vi "ActorLightRun.vi"(8 "ErrorIn":errorcluster, 11 "YActorIn":refnum<class "YActor.lvclass">) -> (0 "ErrorOut":errorcluster, 3 "YActorOut":refnum<class "YActor.lvclass">)   [LabVIEW 2021, in "YActor.lvclass"]
uses:
  YActor.lvclass
  <vilib>/Utility/miscctls.llb/LVPointTypeDef.ctl
  private/ActorPoolFunctions.ctl
  YActor.lvclass/YActor.ctl
  private/GetVIRef.vi
  private/BinaryTracer.vi
  Prefix error msg.vi
  Debug Messages.vi
  private/VIMethodTemplate.vi
  private/RawTrace.vi
panel:
  in  "GuiRef":refnum<vi>
  out "Top Level":string
  in  "LogHistory":u32=30
  out "CommandHistory":string[](array[string])
  in  "KeepOpen":bool
  out "Time Stamp":timestamp format="%<%x %.3X>T"
  in  "SingleStep":bool
  out "Data":string
  out "Command":string
  in  "Continue":bool
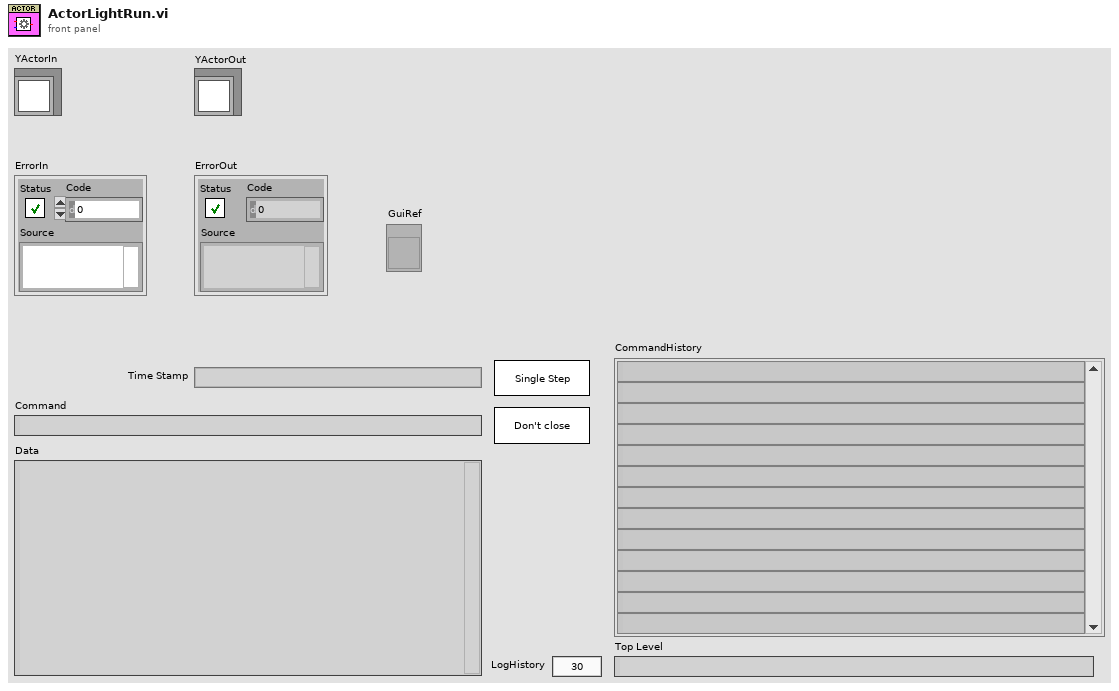
[diagram p1: front panel]
types:
  T1 = typedef "YActor.lvclass/ActorPoolFunctions.ctl" = enum16{"Add", "GetAll", "Delete"}
  T2 = typedef "LVPointTypeDef.ctl" = cluster{"Horizontal":i16, "Vertical":i16}
  T3 = typedef "YActor.lvclass/CmdCtrl.ctl" = cluster{"CmdData":variant, "CommandVI":string, "ReplyQ":i64, "Error":errorcluster, "Msg#":u32, "AsyncErrorHandling":T4, "CallMode":T5, "Source":string}
  T4 = typedef "YActor.lvclass/AsyncErrorHandling.ctl" = enum16{"Return after executing sync command", "Return before executing sync command", "Don't return error"}
  T5 = typedef "YActor.lvclass/CallMode.ctl" = enum16{"Standard", "Call&Collect"}
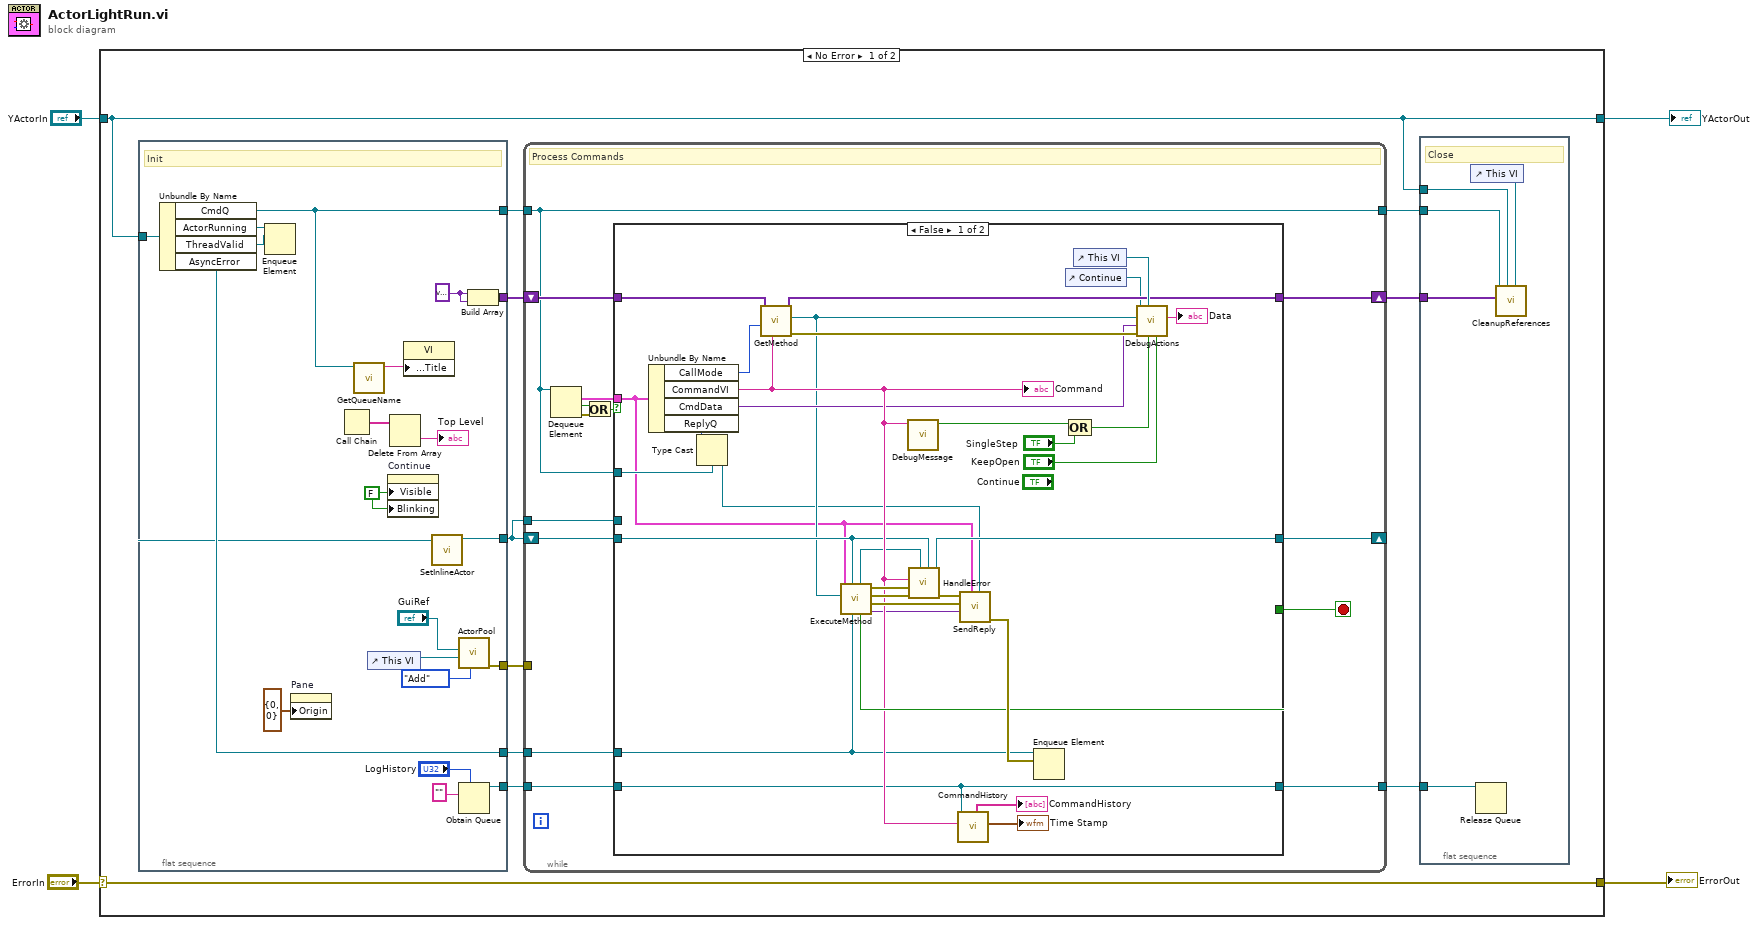
[diagram p0: block diagram]
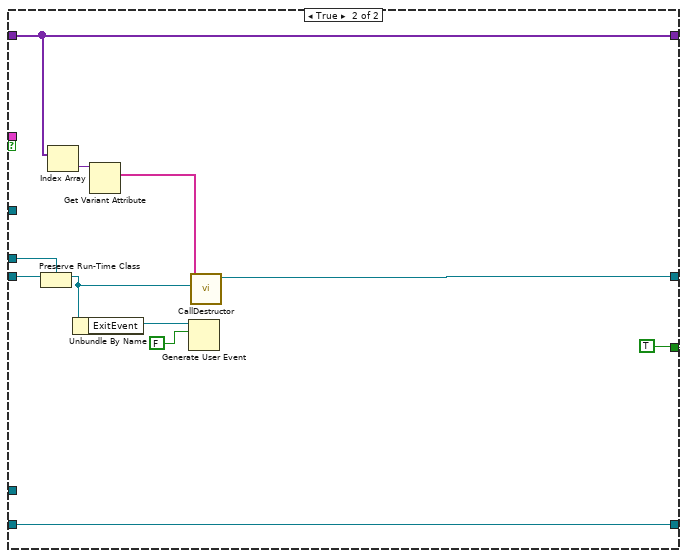
[diagram p2: hidden frame]
diagram:
  n1 = case shown="No Error" "ErrorIn" {
    selector: "ErrorIn" -> [w15 w99]
    tunnel: [w15 w99] -> w3
    tunnel: [w6 w98] -> w1
    tunnel: "YActorIn" -> [w6 w98]
    frame No Error {
      n2 = flat-sequence {
        tunnel: [w21] -> w13
        tunnel: [w37] -> w12
        tunnel: [w35] -> w11
        tunnel: [w29] -> w5
        tunnel: [w27] -> w10
        tunnel: [w40] -> w14
        tunnel: w6 -> [w22]
        frame #0 {
          w28 = variant
          w38 = FALSE ("Visible")
          # "Init"
          n3 = Unbundle By Name(w22) -> ("CmdQ"=w21:refnum<queue>, "ActorRunning"=w33:refnum<queue>, "ThreadValid"=w32:refnum<queue>, "AsyncError"=w27:refnum<queue>)
          n4 = Enqueue Element(queue=w33, element=w32) -> ()  [unwired: 2 in, 3 out]
          n5 = property on="Pane" class="Pane"("Origin"=T2 {"Horizontal"=0, "Vertical"=0}) -> ()  [unwired: 2 in, 2 out]
          n6 = Call Chain() -> (call chain=w31:string[])
          n7 = call "GetQueueName.vi"("QueueIn"=w21) -> ("String"=w26:string)  [unwired: 10 in]
          n8 = control-ref of="This VI"() -> (w24:refnum<vi>)
          n9 = property on="Continue" class="Bool"("Visible"=w38, "Blinking"=w38) -> ()  [unwired: 2 in, 2 out]
          n10 = Delete From Array(array=w31) -> (deleted portion=→"Top Level":string)  [unwired: 2 in, 1 out]
          n11 = property class="VI"("Front Panel.Title"=w26) -> ()  [unwired: 2 in, 2 out]
          n12 = call "SetInlineActor.vi"("YActorIn"=w22) -> ("YActorOut"=w29:refnum<class "YActor.lvclass">)  [unwired: 9 in, 1 out]
          n13 = call "ActorPool.vi"("Functions"=ActorPoolFunctions."Add", "ActorRef"=w24, "GuiRef"="GuiRef") -> ("ErrorOut"=w40:errorcluster)  [unwired: 6 in, 2 out]
          n14 = Obtain Queue(max queue size (-1, unlimited)="LogHistory", element data type="") -> (queue out=w35:refnum<queue>)  [unwired: 3 in, 2 out]
          n15 = Build Array(w28, w28) -> (w37:variant[])
        }
      }
      n16 = while {
        shift-right: [w51] -> w8
        shift-left: w12 -> [w52]
        shift-right: [w50] -> _
        shift-left: w5 -> [w49]
        tunnel: [w41] -> w9
        tunnel: w13 -> [w41]
        tunnel: w11 -> [w45]
        tunnel: w10 -> [w44]
        tunnel: w5 -> [w43]
        tunnel: [w42] -> w7
        tunnel: w14 -> [_]
        stop <- w46 stop-if-true
        # "Process Commands"
        n17 = Dequeue Element(queue=w41) -> (element=w53:T3, timed out?=w48:bool, error out=w54:errorcluster)  [unwired: 2 in, 1 out]
        n18 = Or(x=w48, y=w54) -> (x .or. y?=w47:bool)
        n19 = case shown="False" w47 {
          tunnel: w53 -> [w56 _]
          tunnel: w52 -> [w66 w96]
          tunnel: [w65 w96] -> w51
          tunnel: w41 -> [w80 _]
          tunnel: [w74 w94] -> w50
          tunnel: w49 -> [w61 w95]
          tunnel: [w75 TRUE] -> w46
          tunnel: w45 -> [w57 w87]
          tunnel: w44 -> [w58 _]
          tunnel: w43 -> [_ w93]
          tunnel: [w57 w87] -> w42
          frame False {
            n20 = Unbundle By Name(w56) -> ("CallMode"=w70:T5, "CommandVI"=w71:string, "CmdData"=w63:variant, "ReplyQ"=w79:i64)
            "Command" <- w71
            n21 = Type Cast(type=w80, x=w79) -> (*(type *) &x=w55:refnum<queue>)
            n22 = call "GetMethod.vi"("CommandVI"=w71, "CallMode"=w70, "ReferencesIn"=w66) -> ("ErrorOut"=w86:errorcluster, "VIOut"=w59:refnum<vi>, "ReferencesOut"=w65:variant[])  [unwired: 6 in]
            n23 = call "ExecuteMethod.vi"("AsyncError"=w58, "LabVIEWObjectIn"=w61, "VIIn"=w59, "QueueDataIn"=w56) -> ("ReplyData"=w60:variant, "AsyncErrorOut"=w81:errorcluster, "MethodErrorOut"=w83:errorcluster, "VICallErrorOut"=w84:errorcluster, "Exit"=w75:bool, "LabVIEWObjectOut"=w62:refnum<class>)  [unwired: 2 in]
            n24 = call "DebugMessage.vi"("CommandVI"=w71) -> ("StartDebug"=w76:bool)  [unwired: 10 in]
            n25 = call "HandleError.vi"("LabVIEWObjectIn"=w61, "MethodDataOutput"=w62, "ErrorIn"=w83, "VICallError"=w84, "CommandVI"=w71) -> ("ErrorOut"=w82:errorcluster, "MethodDataOutput"=w74:refnum<class>)  [unwired: 5 in]
            n26 = call "CommandHistory.vi"("CommandVI"=w71, "QueueIn"=w57) -> ("SecondsSince1Jan1904"=→"Time Stamp":timestamp, "HiStory"=→"CommandHistory":string[])  [unwired: 8 in]
            n27 = call "SendReply.vi"("ReplyQueue"=w55, "CmdCtrl"=w56, "ReplyDataIn"=w60, "ASycnErrorIn"=w81, "ErrorIn"=w82) -> ("ErrorOut"=w85:errorcluster)  [unwired: 6 in]
            n28 = Enqueue Element(queue=w58, element=w85) -> ()  [unwired: 2 in, 3 out]
            n29 = control-ref of="Continue"() -> (w64:refnum<vi>)
            n30 = Compound Arithmetic op=OR(w76, "SingleStep") -> (w78:bool)
            n31 = control-ref of="This VI"() -> (w69:refnum<vi>)
            n32 = call "DebugActions.vi"("KeepOpen"="KeepOpen", "DebugOn"=w78, "ThisVI"=w69, "ErrorIn"=w86, "CmdData"=w63, "VIIn"=w59, "Continue"=w64) -> ("XmlString"=→"Data":string)  [unwired: 3 in, 1 out]
          }
          frame True {
            n33 = Preserve Run-Time Class(object in=w95, 2:w93) -> (object out=w88:refnum<class "YActor.lvclass">)  [unwired: 1 in, 1 out]
            n34 = Index Array(array=w96) -> (element=w90:variant)  [unwired: 1 in]
            n35 = Unbundle By Name(w88) -> ("ExitEvent"=w92:refnum<user-event>)
            n36 = Get Variant Attribute(Variant=w90) -> (names=w89:string[])  [unwired: 3 in, 3 out]
            n37 = Generate User Event(user event=w92, event data cluster=FALSE ("event data")) -> ()  [unwired: 2 in, 2 out]
            n38 = call "CallDestructor.vi"("ActorLightIn"=w88, "Array"=w89) -> ("YActorOut"=w94:refnum<class>)  [unwired: 9 in]
          }
        }
      }
      n39 = flat-sequence {
        tunnel: w9 -> [w20]
        tunnel: w8 -> [w19]
        tunnel: w7 -> [w17]
        tunnel: w6 -> [w16]
        frame #0 {
          # "Close"
          n40 = control-ref of="This VI"() -> (w18:refnum<vi>)
          n41 = Release Queue(queue=w17) -> ()  [unwired: 2 in, 3 out]
          n42 = call "CleanupReferences.vi"("ActorRef"=w18, "ActorLightIn"=w16, "ArrayIn"=w19, "CmdQ"=w20) -> ()  [unwired: 8 in]
        }
      }
    }
    frame Error {
    }
  }
  "ErrorOut" <- w3
  "YActorOut" <- w1
